vi "Simple Example.vi"() -> ()   [LabVIEW 2017]
uses:
  Handler.UserEvent.Console/Handler.UserEvent.Console.lvclass
  \\192.168.1.40\Neosoft/Partage/Dossiers Personnels/BRO/DevTools_BR/wc/ErrorLog/src/Handler/Handler.lvclass
  Handler.File.Text/Handler.File.Text.lvclass
  Logger/Logger.lvclass
panel:
  in  "Error Message":string="Error log message."
  in  "Error":errorcluster={"status"=TRUE, "code"=5000, "source"="My Error Code"}
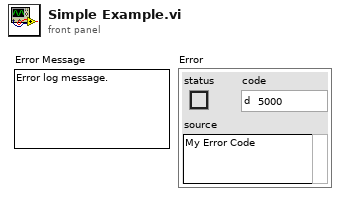
[diagram p1: front panel]
types:
  T1 = enum16{"DEBUG", "INFO", "WARNING", "ERROR", "CRITICAL"}
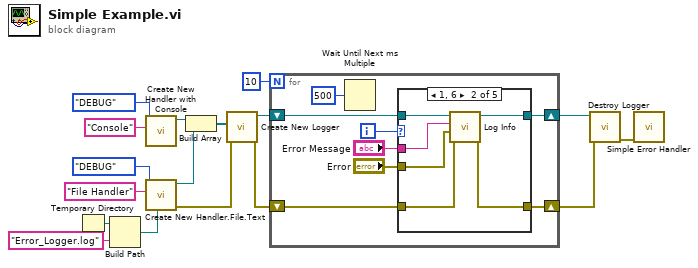
[diagram p0: block diagram]
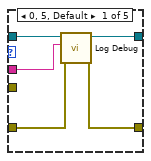
[diagram p2: hidden frame]
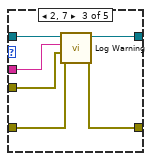
[diagram p3: hidden frame]
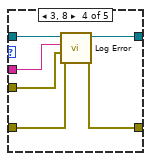
[diagram p4: hidden frame]
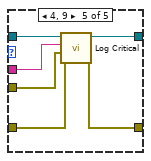
[diagram p5: hidden frame]
diagram:
  n1 = Temporary Directory() -> (w13:path)
  n2 = Build Path(base path=w13, name or relative path="Error_Logger.log") -> (appended path=w11:path)
  n3 = call "Create New Handler with Console.vi"("Name"="Console", "Level"=T1."DEBUG") -> ("Handler.UserEvent.Console out"=w3:refnum<class "Handler.UserEvent.Console.lvclass">)  [unwired: 8 in, 1 out]
  n4 = call "Create New Handler.File.Text.vi"("File Path"=w11, "Name"="File Handler", "Level"=T1."DEBUG") -> ("error out"=w4:errorcluster, "Handler.File.Text out"=w10:refnum<class "Handler.File.Text.lvclass">)  [unwired: 7 in]
  n5 = Build Array(w3, w10) -> (w17:refnum<class "Handler.lvclass">[])
  n6 = call "Create New Logger.vi"("error in (no error)"=w4, "Handlers"=w17) -> ("error out"=w9:errorcluster, "Logger out"=w16:refnum<class "Logger.lvclass">)  [unwired: 8 in]
  n7 = for {
    N: 10 -> [_]
    shift-right: [w21] -> w7
    shift-left: w16 -> [w22]
    shift-right: [w20] -> w6
    shift-left: w9 -> [w23]
    i -> [w18]
    n8 = Wait Until Next ms Multiple(millisecond multiple=u32 500) -> ()  [unwired: 1 out]
    n9 = case shown="1, 6" w18 {
      tunnel: w22 -> [w30 w36 w42 w48 w54]
      tunnel: [w29 w35 w41 w47 w53] -> w21
      tunnel: w23 -> [w28 w34 w40 w46 w52]
      tunnel: [w27 w33 w39 w45 w51] -> w20
      tunnel: "Error Message" -> [w26 w32 w38 w44 w50]
      tunnel: "Error" -> [_ w31 w37 w43 w49]
      frame 0, 5, Default {
        n10 = call "Log Debug.vi"("error in (no error)"=w28, "Message"=w26, "Logger in"=w30) -> ("error out"=w27:errorcluster, "Logger out"=w29:refnum<class "Logger.lvclass">)  [unwired: 7 in]
      }
      frame 1, 6 {
        n11 = call "Log Info.vi"("error in (no error)"=w34, "error"=w31, "Message"=w32, "Logger in"=w36) -> ("error out"=w33:errorcluster, "Logger out"=w35:refnum<class "Logger.lvclass">)  [unwired: 6 in]
      }
      frame 2, 7 {
        n12 = call "Log Warning.vi"("error in (no error)"=w40, "error"=w37, "Message"=w38, "Logger in"=w42) -> ("error out"=w39:errorcluster, "Logger out"=w41:refnum<class "Logger.lvclass">)  [unwired: 6 in]
      }
      frame 3, 8 {
        n13 = call "Log Error.vi"("error in (no error)"=w46, "error"=w43, "Message"=w44, "Logger in"=w48) -> ("error out"=w45:errorcluster, "Logger out"=w47:refnum<class "Logger.lvclass">)  [unwired: 6 in]
      }
      frame 4, 9 {
        n14 = call "Log Critical.vi"("error in (no error)"=w52, "error"=w49, "Message"=w50, "Logger in"=w54) -> ("error out"=w51:errorcluster, "Logger out"=w53:refnum<class "Logger.lvclass">)  [unwired: 6 in]
      }
    }
  }
  n15 = call "Destroy Logger.vi"("error in (no error)"=w6, "Logger in"=w7) -> ("error out"=w5:errorcluster)  [unwired: 8 in, 1 out]
  n16 = call <vilib>:"Simple Error Handler.vi"("error in (no error)"=w5) -> ()  [unwired: 4 in, 5 out]
